vi "AKM43L_InitParam.vi"(0 "PID Loop Period":dbl=0.001 format="%#_13g", 1 "Motor Quantity":i32=8, 3 "error in (no error)":errorcluster) -> (7 "MotorCtrl":refnum<class "MotorControl.lvclass">, 10 "error out":errorcluster)   [LabVIEW 2015, in "AKM43L.lvclass"]
uses:
  AKM43L.lvclass
  MotorControl/MotorControl.lvclass
panel:
  in  "PID gain schedule":T1(array[cluster])=[[{"PID gains"={"proportional gain (Kc)"=0.03, "integral time (Ti, min)"=0.000783, "derivative time (Td, min)"=0.0002}, "max value"=0.0}, {"PID gains"={"proportional gain (Kc)"=0.05, "integral time (Ti, min)"=0.000783, "derivative time (Td, min)"=0.0002}, "max value"=100.0}]]
  in  "FrictionModel":cluster{"Coeff+":dbl[], "Coeff-":dbl[]}
  in  "MotorConstant(F/V)":dbl=43.0
  in  "Force Rate (N/min)":cluster{"ForceRateLow":dbl, "ForceRateHigh":dbl}={"ForceRateLow"=300.0, "ForceRateHigh"=60000.0} {"ForceRateHigh" format="%#_13g"; "ForceRateLow" format="%#_13g"}
  in  "TransferRatio":dbl=1.0 format="%#_13g"
  in  "output range":cluster{"output high":dbl, "output low":dbl}={"output high"=5.0, "output low"=-0.5}
  in  "setpoint range":cluster{"setpoint high":dbl, "setpoint low":dbl}={"setpoint high"=100.0, "setpoint low"=5.0}
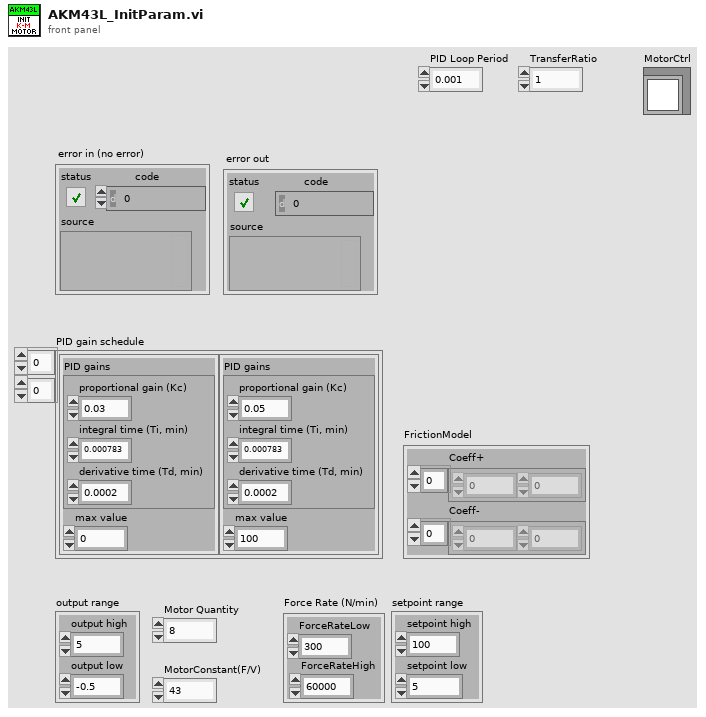
[diagram p1: front panel]
types:
  T1 = cluster{"PID gains":cluster{"proportional gain (Kc)":dbl, "integral time (Ti, min)":dbl, "derivative time (Td, min)":dbl}, "max value":dbl}[][]
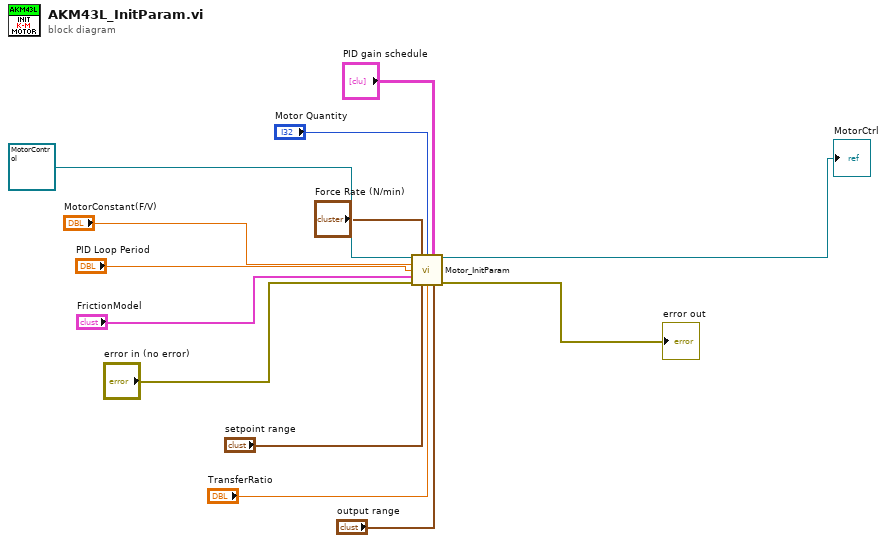
[diagram p0: block diagram]
diagram:
  n1 = call "Motor_InitParam.vi"("Motor Control In"=refnum<class "MotorControl.lvclass"> refnum ("MotorCtrl_In"), "Force Rate Limit (N/min)"="Force Rate (N/min)", "Motor Quantity"="Motor Quantity", "PID gain schedule"="PID gain schedule", "MotorConstant(F/V)"="MotorConstant(F/V)", "PID Loop Period"="PID Loop Period", "FrictionModel"="FrictionModel", "error in (no error)"="error in (no error)", "output range (N)"="setpoint range", "TransferRatio"="TransferRatio", "setpoint range (A)"="output range") -> ("Motor Control Out"=→"MotorCtrl":refnum<class "MotorControl.lvclass">, "error out"=→"error out":errorcluster)  [unwired: 3 in]
